vi "Config CDMA2000 Forward.vi"(0 "VISA Resource Name":refnum<visa-resource-name>, 1 "Forward Select (3: S1 9 Channel)":T2(ring)=enum."S1 9 Channel", 2 "Custom State File (CDMA_DATA)":string="CDMA_DATA", 4 "Reconstruction Filter (1:2.5MHZ)":T1(ring)=enum."2.5 MHZ", 5 "error in (no error)":errorcluster {"code" format="%.0x"}, 7 "Multicarrier (0: CAR2)":enum16{"CAR2", "CAR3", "CAR4", "CUSTOM"}(ring), 10 "ARB Reference (F:INT)":bool, 12 "Reference Freq (10.0)":dbl=10.0 format="%.8f") -> (14 "VISA Resource Name Out":refnum<visa-resource-name>, 19 "error out":errorcluster {"code" format="%.0x"})   [LabVIEW 2014, in "Agilent ESG Series.lvlib"]
doc: "This VI is used to configure the forward CDMA2000 option.\n\nNotes:\nThis VI is valid only on instruments E44xxB with the 101 option or on instrument E4438C with option 401."
uses:
  Agilent ESG Series.lvlib
panel:
  # "EXT"
  # "INT"
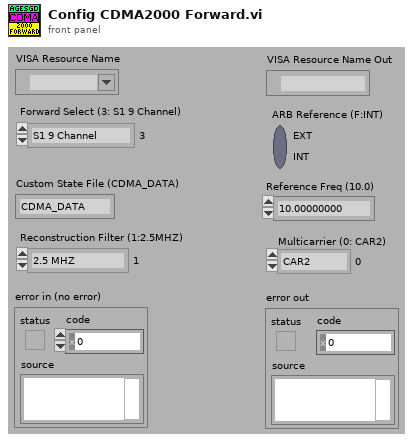
[diagram p1: front panel]
types:
  T1 = enum16{"250 KHZ", "2.5 MHZ", "8.0 MHZ", "THROUGH"}
  T2 = enum16{"S1 Pilot", "S3D Pilot", "S3M Pilot", "S1 9 Channel", "S3D 9 Channel", "S3M 9 Channel", "Custom", "Multicarrier"}
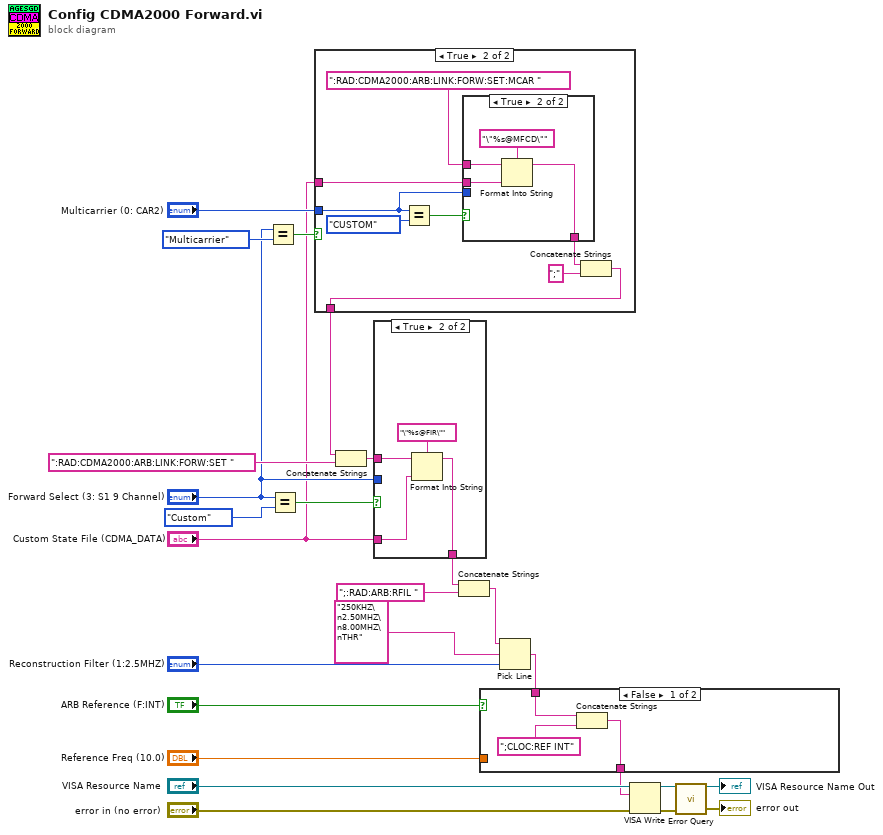
[diagram p0: block diagram]
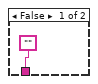
[diagram p2: hidden frame]
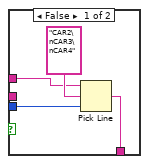
[diagram p3: hidden frame]
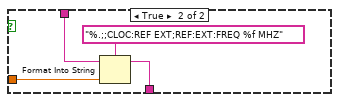
[diagram p4: hidden frame]
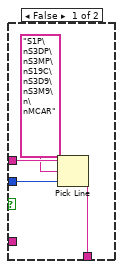
[diagram p5: hidden frame]
diagram:
  n1 = Equal?(x="Forward Select (3: S1 9 Channel)", y=T2."Multicarrier" ("Forward Select (3: S1 9 Channel)")) -> (x = y?=w4:bool)
  n2 = Equal?(x="Forward Select (3: S1 9 Channel)", y=T2."Custom" ("Forward Select (3: S1 9 Channel)")) -> (x = y?=w22:bool)
  n3 = case shown="True" w4 {
    tunnel: "Multicarrier (0: CAR2)" -> [_ w27]
    tunnel: "Custom State File (CDMA_DATA)" -> [_ w31]
    tunnel: ["" w28] -> w1
    frame False {
    }
    frame True {
      n4 = Equal?(x=w27, y=enum16{"CAR2", "CAR3", "CAR4", "CUSTOM"}."CUSTOM" ("Multicarrier (0: CAR2)")) -> (x = y?=w32:bool)
      n5 = case shown="True" w32 {
        tunnel: [w37 w41] -> w30
        tunnel: ":RAD:CDMA2000:ARB:LINK:FORW:SET:MCAR " ("string (\"\")") -> [w36 w40]
        tunnel: w31 -> [_ w39]
        tunnel: w27 -> [w35 _]
        frame False {
          n6 = Pick Line(string ("")=w36, multi-line string="CAR2\nCAR3\nCAR4", line index=w35) -> (output string=w37:string)
        }
        frame True {
          n7 = Format Into String(format string="\"%s@MFCD\"", initial string=w40, w39) -> (resulting string=w41:string)  [unwired: 1 in, 1 out]
        }
      }
      n8 = Concatenate Strings(w30, ";") -> (w28:string)
    }
  }
  n9 = Concatenate Strings(w1, ":RAD:CDMA2000:ARB:LINK:FORW:SET " ("string (\"\")")) -> (w8:string)
  n10 = case shown="True" w22 {
    tunnel: w8 -> [w46 w50]
    tunnel: "Forward Select (3: S1 9 Channel)" -> [w44 _]
    tunnel: [w43 w48] -> w9
    tunnel: "Custom State File (CDMA_DATA)" -> [_ w47]
    frame False {
      n11 = Pick Line(string ("")=w46, multi-line string="S1P\nS3DP\nS3MP\nS19C\nS3D9\nS3M9\n\nMCAR", line index=w44) -> (output string=w43:string)
    }
    frame True {
      n12 = Format Into String(format string="\"%s@FIR\"", initial string=w50, w47) -> (resulting string=w48:string)  [unwired: 1 in, 1 out]
    }
  }
  n13 = Concatenate Strings(w9, ";:RAD:ARB:RFIL " ("string (\"\")")) -> (w18:string)
  n14 = Pick Line(string ("")=w18, multi-line string="250KHZ\n2.50MHZ\n8.00MHZ\nTHR", line index="Reconstruction Filter (1:2.5MHZ)") -> (output string=w19:string)
  n15 = case shown="False" "ARB Reference (F:INT)" {
    tunnel: w19 -> [w53 w57]
    tunnel: [w51 w54] -> w14
    tunnel: "Reference Freq (10.0)" -> [_ w55]
    frame False {
      n16 = Concatenate Strings(w53, ";CLOC:REF INT") -> (w51:string)
    }
    frame True {
      n17 = Format Into String(format string="%.;;CLOC:REF EXT;REF:EXT:FREQ %f MHZ", initial string=w57, w55) -> (resulting string=w54:string)  [unwired: 1 in, 1 out]
    }
  }
  n18 = VISA Write(VISA resource name="VISA Resource Name", write buffer=w14, error in (no error)="error in (no error)") -> (VISA resource name out=w13:refnum<visa-resource-name>, error out=w12:errorcluster)  [unwired: 1 out]
  n19 = call "Error Query.vi"("VISA Resource Name"=w13, "error in (no error)"=w12) -> ("VISA Resource Name Out"=→"VISA Resource Name Out":refnum<visa-resource-name>, "error out"=→"error out":errorcluster)  [unwired: 10 in, 2 out]
